vi "timestampOffset.vi"(10 "Reference Time":timestamp) -> (2 "Timestamp Offset":ext)   [LabVIEW 2013, in "Epoch.lvclass"]
uses:
  Epoch.lvclass
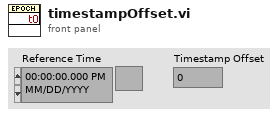
[diagram p1: front panel]
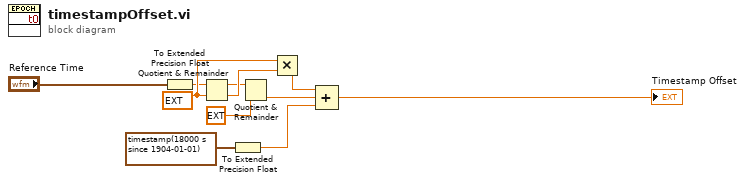
[diagram p0: block diagram]
diagram:
  w5 = ext 3600.0 ("y")
  n1 = To Extended Precision Float(1:"Reference Time") -> (0:w3:ext)
  n2 = Quotient & Remainder(x=w3, y=w5) -> (x-y*floor(x/y)=w2:ext, floor(x/y)=w6:ext)
  n3 = To Extended Precision Float(1:timestamp(18000 s since 1904-01-01) ("current time")) -> (0:w8:ext)
  n4 = Quotient & Remainder(x=w2, y=ext 60.0) -> (floor(x/y)=w9:ext)  [unwired: 1 out]
  n5 = Multiply(x=w5, y=w6) -> (x*y=w10:ext)
  n6 = Compound Arithmetic op=ADD(w10, w9, w8) -> (→"Timestamp Offset":ext)
